vi "DAQ_ADC_Max_Sample_Rate_For_USB_6001.vi"(8 "error in":errorcluster, 10 "number of samples per channel":i32=10000, 11 "Refnum in":refnum<k21>) -> (0 "error out":errorcluster, 3 "data":waveform(dbl))   [LabVIEW 2017]
uses:
  <vilib>/DAQmx/read.llb/DAQmx Read (Analog Wfm 1Chan NSamp).vi
  <vilib>/DAQmx/miscellaneous.llb/DAQmx Fill In Error Info.vi
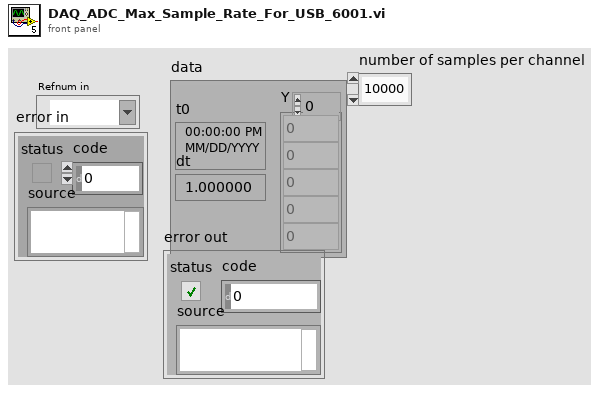
[diagram p1: front panel]
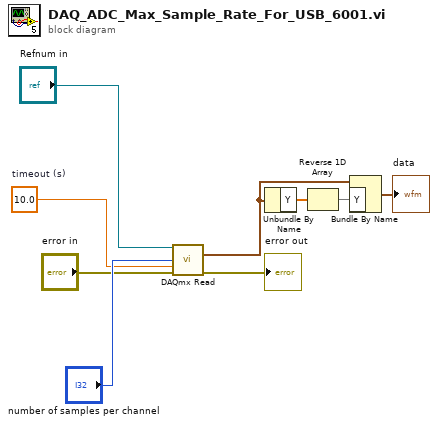
[diagram p0: block diagram]
diagram:
  w3 = 10.0  # timeout (s)
  n1 = call-poly <vilib>:"DAQmx Read.vi"("task/channels in"="Refnum in", "number of samples per channel"="number of samples per channel", "timeout"=w3, "error in"="error in") -> ("data"=w8:waveform(dbl), "error out"=→"error out":errorcluster)  [unwired: 9 in, 1 out]
  n2 = Unbundle By Name(w8) -> ("Y"=w6:dbl[])
  n3 = Reverse 1D Array(array=w6) -> (reversed array=w9:dbl[])
  n4 = Bundle By Name(cluster=w8, "Y"=w9) -> (→"data":waveform(dbl))
